vi "ComputeCoeffcients_vg.vi"(9 "k-constant":dbl=3.01, 11 "Numeric":i32=32) -> (1 "cosine":i16[](array[numeric])=[71, 0, -71, -100, -71, 0, 71, 100, 71, 0, -71, -100, -71, 0, 71, 100, 71, 0, -71, -100, -71, 0, 71, 100, 71, 0, -71, -100, -71, 0, 71, 100], 3 "sine":i16[](array[numeric])=[71, 100, 71, 0, -71, -100, -71, 0, 71, 100, 71, 0, -71, -100, -71, 0, 71, 100, 71, 0, -71, -100, -71, 0, 71, 100, 71, 0, -71, -100, -71, 0])   [LabVIEW 2020]
panel:
  out "Waveform Chart 2":i16[](graph)=[71, 0, -71, -100, -71, 0, 71, 100, 71, 0, -71, -100, -71, 0, 71, 100, 71, 0, -71, -100, -71, 0, 71, 100, 71, 0, -71, -100, -71, 0, 71, 100]
  out "Waveform Chart":i16[](graph)=[71, 100, 71, 0, -71, -100, -71, 0, 71, 100, 71, 0, -71, -100, -71, 0, 71, 100, 71, 0, -71, -100, -71, 0, 71, 100, 71, 0, -71, -100, -71, 0]
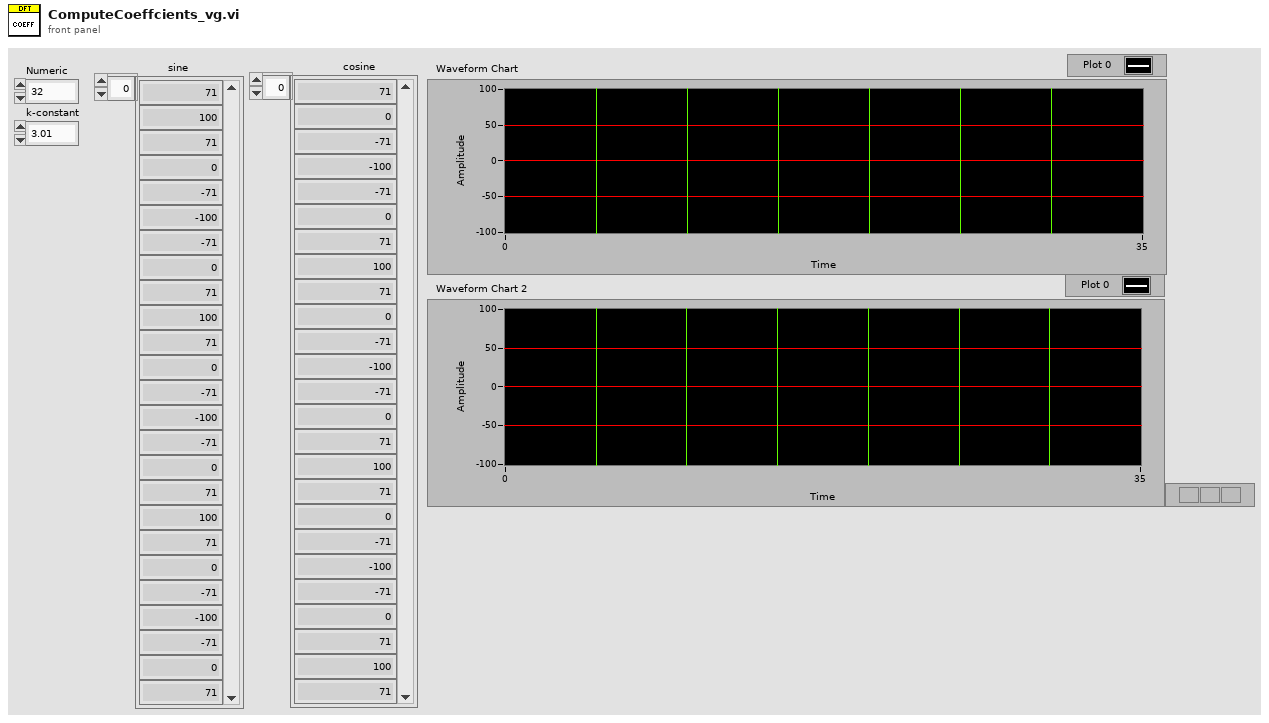
[diagram p1: front panel]
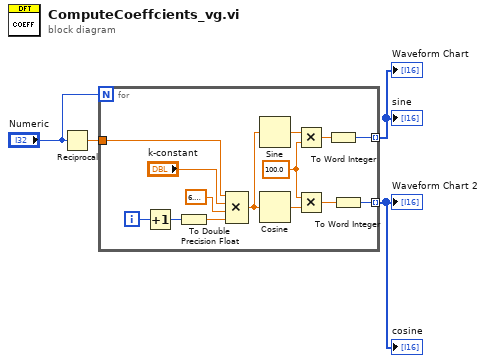
[diagram p0: block diagram]
diagram:
  n1 = Reciprocal(x="Numeric") -> (1/x=w3:dbl)
  n2 = for {
    N: "Numeric" -> [_]
    tunnel: w3 -> [w14]
    tunnel: [w6] -> w1 mode=indexing
    tunnel: [w5] -> w2 mode=indexing
    i -> [w16]
    w10 = 100.0 ("y")
    n3 = Increment(x=w16) -> (x+1=w13:i32)
    n4 = To Double Precision Float(number=w13) -> (double precision float=w15:dbl)
    n5 = Compound Arithmetic op=MULTIPLY(w14, "k-constant", 6.283185307179586, w15) -> (w12:dbl)
    n6 = Sine(x=w12) -> (sin(x)=w11:dbl)
    n7 = Cosine(x=w12) -> (cos(x)=w9:dbl)
    n8 = Multiply(x=w11, y=w10) -> (x*y=w8:dbl)
    n9 = Multiply(x=w10, y=w9) -> (x*y=w7:dbl)
    n10 = To Word Integer(number=w8) -> (16bit integer=w6:i16)
    n11 = To Word Integer(number=w7) -> (16bit integer=w5:i16)
  }
  "sine" <- w1
  "cosine" <- w2
  "Waveform Chart" <- w1
  "Waveform Chart 2" <- w2
